vi "SetSpriteActive.vi"(8 "error in (no error)":errorcluster, 9 "Active":bool, 10 "index":i16, 11 "Game in":refnum<class "Game.lvclass">) -> (0 "error out":errorcluster, 3 "Game out":refnum<class "Game.lvclass">)   [LabVIEW 2019, in "RT_Game.lvlib" / "Game.lvclass"]
uses:
  Game.lvclass
  Game.lvclass/Game.ctl
  GameObject/GameObject.lvclass/GameObject.ctl
  GameObject/Write IsActive.vi
  RT_Sprite/RT_Sprite.lvclass
  C:/Users/FreshBob/Dropbox/VIs/myRIO_GameConsole/RT/RT_Game/GameObject/GameObject.lvclass
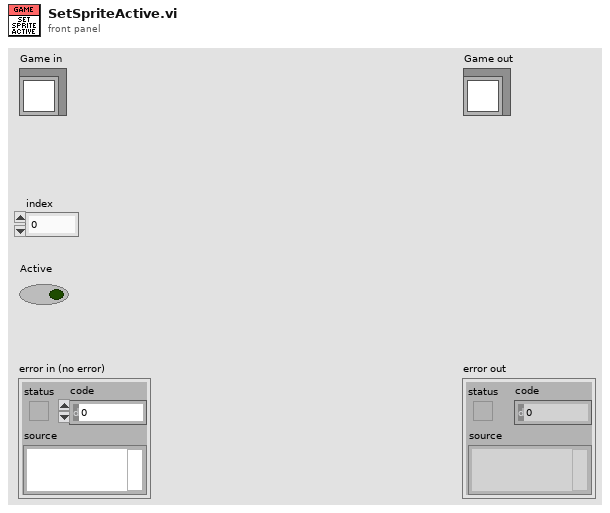
[diagram p1: front panel]
types:
  T1 = typedef "RT_Game.lvlib/Game.lvclass/SpritesCluster.ctl" = cluster{"Sprite1":refnum<class "RT_Sprite.lvclass">, "Sprite2":refnum<class "RT_Sprite.lvclass">, "Sprite3":refnum<class "RT_Sprite.lvclass">}
  T2 = cluster{"Sprites[0]":refnum<class "RT_Sprite.lvclass">, "Sprites[1]":refnum<class "RT_Sprite.lvclass">, "Sprites[2]":refnum<class "RT_Sprite.lvclass">}
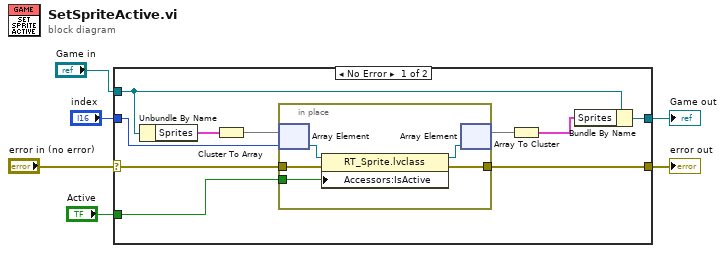
[diagram p0: block diagram]
diagram:
  n1 = case shown="No Error" "error in (no error)" {
    selector: "error in (no error)" -> [w11 w23]
    tunnel: [w10 w23] -> w5
    tunnel: [w13 w22] -> w3
    tunnel: "Game in" -> [w16 w22]
    tunnel: "index" -> [w14 _]
    tunnel: "Active" -> [w9 _]
    frame No Error {
      n2 = Unbundle By Name(w16) -> ("Sprites"=w15:T1)
      n3 = Cluster To Array(cluster=w15) -> (array=w8:refnum<class "RT_Sprite.lvclass">[])
      n4 = in-place {
        in-place-border: [w20] -> w10
        in-place-border: w11 -> [w21]
        in-place-border: w9 -> [w17]
        n5 = in-place-array #1(w8, w14) -> (w19:refnum<class "RT_Sprite.lvclass">)
        n6 = property class="RT_Sprite.lvclass"(reference=w19, error in=w21, "Accessors:IsActive"=w17) -> (reference out=w18:refnum<class "RT_Sprite.lvclass">, error out=w20:errorcluster)
        n7 = in-place-array #1(w18) -> (w12:refnum<class "RT_Sprite.lvclass">[])  [unwired: 1 out]
      }
      n8 = Array To Cluster(array=w12) -> (cluster=w7:T2)
      n9 = Bundle By Name(cluster=w16, "Sprites"=w7) -> (w13:refnum<class "Game.lvclass">)
    }
    frame Error {
    }
  }
  "error out" <- w5
  "Game out" <- w3
